vi "Construct Open VIPM Step.vi"(5 "Open VIPM Step in":refnum<class "Open VIPM Step.lvclass">, 8 "error in (no error)":errorcluster) -> (0 "error out":errorcluster, 3 "Open VIPM Step":refnum<class "Open VIPM Step.lvclass">)   [LabVIEW 2019, in "VIPM.lvlib" / "Open VIPM Step.lvclass"]
uses:
  Open VIPM Step.lvclass
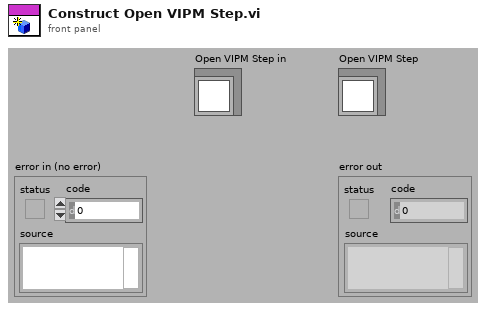
[diagram p1: front panel]
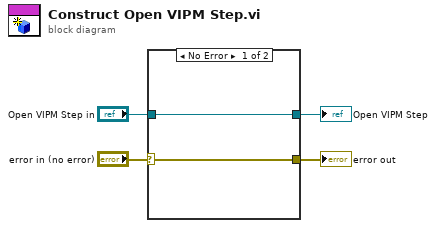
[diagram p0: block diagram]
diagram:
  n1 = case shown="No Error" "error in (no error)" {
    selector: "error in (no error)" -> [w6 w8]
    tunnel: [w6 w8] -> w3
    tunnel: [w5 w7] -> w1
    tunnel: "Open VIPM Step in" -> [w5 w7]
    frame No Error {
    }
    frame Error {
    }
  }
  "error out" <- w3
  "Open VIPM Step" <- w1
